vi "register new subscription.vi"(9 "communicator":refnum<class "communicator.lvclass">, 10 "pattern":string, 11 "registered subscriptions in":T1) -> (3 "registered subscriptions out":T1)   [LabVIEW 2015, in "publisher.lvclass"]
uses:
  publisher.lvclass
  registered subscriptions.ctl
  communicator/communicator.lvclass
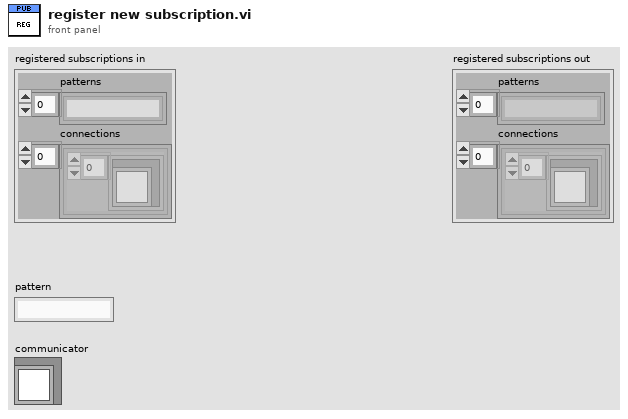
[diagram p1: front panel]
types:
  T1 = typedef "publisher.lvclass/registered subscriptions.ctl" = cluster{"patterns":string[], "connections":cluster{"connections":refnum<class "communicator.lvclass">[]}[]}
  T2 = cluster{"connections":refnum<class "communicator.lvclass">[]}[]
  T3 = cluster{"connections":refnum<class "communicator.lvclass">[]}
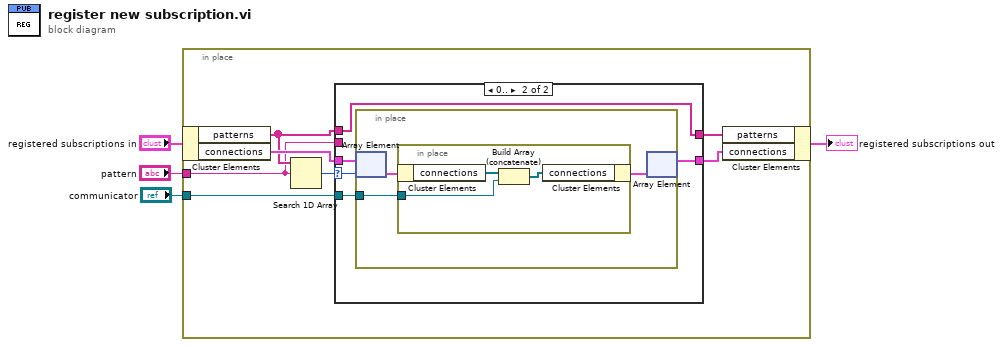
[diagram p0: block diagram]
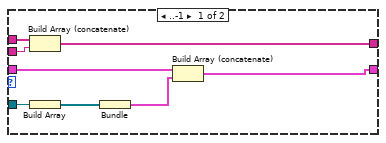
[diagram p2: hidden frame]
diagram:
  n1 = in-place {
    in-place-border: "pattern" -> [w5]
    in-place-border: "communicator" -> [w6]
    n2 = in-place-cluster #1("registered subscriptions in") -> ("patterns"=w8:string[], "connections"=w10:T2)
    n3 = Search 1D Array(1D array=w8, element=w5) -> (index of element=w11:i32)  [unwired: 1 in]
    n4 = case shown="0.." w11 {
      selector: w11 -> [_ w21]
      tunnel: w10 -> [w19 w24]
      tunnel: [w18 w23] -> w9
      tunnel: w8 -> [w16 w22]
      tunnel: [w17 w22] -> w7
      tunnel: w6 -> [w14 w20]
      tunnel: w5 -> [w15 _]
      frame ..-1 {
        n5 = Build Array (concatenate)(w16, w15) -> (w17:string[])
        n6 = Build Array(w14) -> (w13:refnum<class "communicator.lvclass">[])
        n7 = Bundle(w13) -> (w12:cluster{refnum<class "communicator.lvclass">[]})  [unwired: 1 in]
        n8 = Build Array (concatenate)(w19, w12) -> (w18:T2)
      }
      frame 0.. {
        n9 = in-place {
          in-place-border: w20 -> [w25]
          n10 = in-place-array #2(w24, w21) -> (w27:T3)
          n11 = in-place {
            in-place-border: w25 -> [w28]
            n12 = in-place-cluster #3(w27) -> ("connections"=w30:refnum<class "communicator.lvclass">[])
            n13 = Build Array (concatenate)(w30, w28) -> (w29:refnum<class "communicator.lvclass">[])
            n14 = in-place-cluster #3("connections"=w29) -> (w26:T3)
          }
          n15 = in-place-array #2(w26) -> (w23:T2)  [unwired: 1 out]
        }
      }
    }
    n16 = in-place-cluster #1("patterns"=w7, "connections"=w9) -> (→"registered subscriptions out":T1)
  }
